vi "CRYPlot Graph Sub.vi"(9 "nData2 In":i32[](array[numeric]), 10 "nData1 In":i32[](array[numeric]), 11 "Type":enum16{"Curves", "Values", "Results", "WFM"}(ring)) -> (2 "nData Out":i32[](array[numeric]))   [LabVIEW 2013]
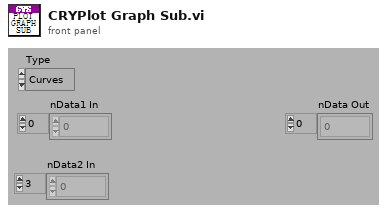
[diagram p1: front panel]
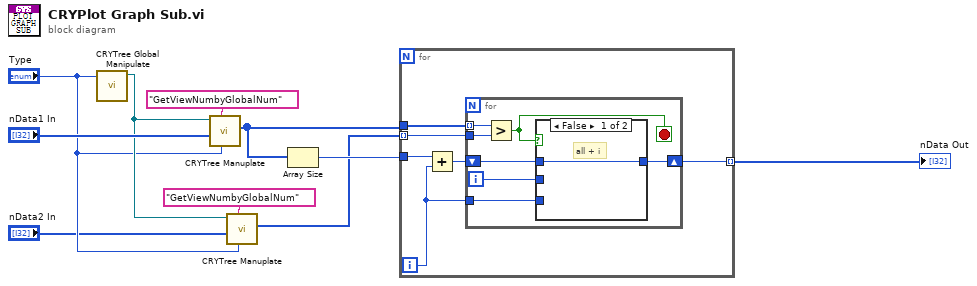
[diagram p0: block diagram]
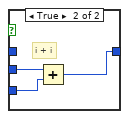
[diagram p2: hidden frame]
diagram:
  n1 = call "CRYTree Global Manipulate.vi"("Type In"="Type") -> ("Tree/Curve Tree"=w4:refnum<vi>)  [unwired: 7 in, 3 out]
  n2 = call "CRYTree Manuplate.vi"("Type"="Type", "sAction"="GetViewNumbyGlobalNum", "nData"="nData1 In", "Tree in"=w4) -> ("nData Out"=w6:i32[])  [unwired: 4 in, 3 out]
  n3 = call "CRYTree Manuplate.vi"("Type"="Type", "sAction"="GetViewNumbyGlobalNum", "nData"="nData2 In", "Tree in"=w4) -> ("nData Out"=w1:i32[])  [unwired: 4 in, 3 out]
  n4 = Array Size(array=w6) -> (size(s)=w10:i32)
  n5 = for {
    tunnel: w1 -> [w15] mode=indexing
    tunnel: w6 -> [w16]
    tunnel: w10 -> [w14]
    tunnel: [w11] -> w9 mode=indexing
    i -> [w12]
    n6 = Add(x=w14, y=w12) -> (x+y=w13:i32)
    n7 = for {
      tunnel: w16 -> [w23] mode=indexing
      tunnel: w15 -> [w22]
      shift-right: [w20] -> w11
      shift-left: w13 -> [w19]
      tunnel: w12 -> [w17]
      i -> [w21]
      stop <- w18 stop-if-true
      n8 = Greater?(x=w23, y=w22) -> (0:w18:bool)
      n9 = case shown="False" w18 {
        tunnel: w21 -> [_ w27]
        tunnel: [w24 w25] -> w20
        tunnel: w19 -> [w24 _]
        tunnel: w17 -> [_ w26]
        frame False {
          # "all + i"
        }
        frame True {
          # "i + i"
          n10 = Add(x=w27, y=w26) -> (x+y=w25:i32)
        }
      }
    }
  }
  "nData Out" <- w9
